vi "matlab_TI2_lightpath.vi"(8 "error in":errorcluster, 10 "Lightpath":u16(ring) items=["1-EYE", "2-R100", "3-AUX", "4-L100"]) -> (0 "error out":errorcluster)   [LabVIEW 2018]
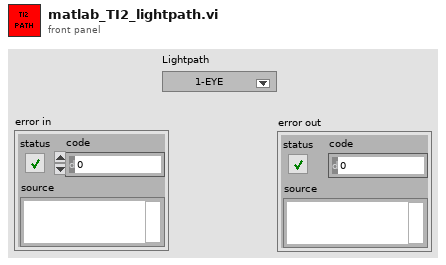
[diagram p1: front panel]
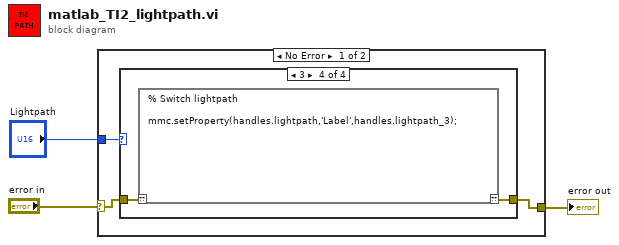
[diagram p0: block diagram]
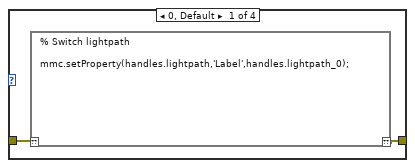
[diagram p2: hidden frame]
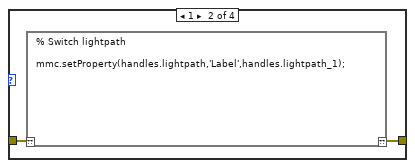
[diagram p3: hidden frame]
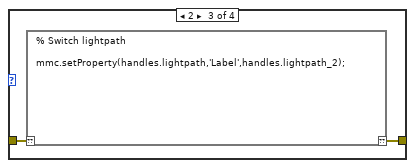
[diagram p4: hidden frame]
diagram:
  n1 = case shown="No Error" "error in" {
    selector: "error in" -> [w5 w15]
    tunnel: [w4 w15] -> w2
    tunnel: "Lightpath" -> [w6 _]
    frame No Error {
      n2 = case shown="3" w6 {
        tunnel: w5 -> [w8 w10 w12 w14]
        tunnel: [w7 w9 w11 w13] -> w4
        frame 0, Default {
          n3 = script code="% Switch lightpath\n\nmmc.setProperty(handles.lightpath,'Label',handles.lightpath_0);"("??"=w8) -> ("??"=w7:errorcluster)
        }
        frame 1 {
          n4 = script code="% Switch lightpath\n\nmmc.setProperty(handles.lightpath,'Label',handles.lightpath_1);"("??"=w10) -> ("??"=w9:errorcluster)
        }
        frame 2 {
          n5 = script code="% Switch lightpath\n\nmmc.setProperty(handles.lightpath,'Label',handles.lightpath_2);"("??"=w12) -> ("??"=w11:errorcluster)
        }
        frame 3 {
          n6 = script code="% Switch lightpath\n\nmmc.setProperty(handles.lightpath,'Label',handles.lightpath_3);"("??"=w14) -> ("??"=w13:errorcluster)
        }
      }
    }
    frame Error {
    }
  }
  "error out" <- w2
